vi "HEWH Get SUf Index.vi"(7 "Water Heater Type":T6, 8 "error in (no error)":errorcluster, 11 "UEF Calculated Values":T1={"Calculated Values"={"Draw Cluster - Actual (Gal)"=[], "Mass of water All (lbm)"=[], "Density of hot water All (lbm/gal)"=[], "CpHW (BTU/(lbm °F))"=[], "rho 2 (lb/gal)"=0.0, "rho standby (lb/gal)"=0.0, "rho 24 (lb/gal)"=0.0, "Cp1 (BTU/(lb*F))"=0.0, "Cp2 (BTU/(lb*F))"=0.0, "Cp standby (BTU/(lb*F))"=0.0, "Cp 24 (BTU/(lb*F))"=0.0, "nu_r"=0.0, "Qstby (BTU)"=0.0, "Qhr (BTU/hr)"=0.0, "UA (BTU/(hr*F))"=0.0, "Q (BTU)"=0.0, "Qd (BTU)"=0.0, "Qda (BTU)"=0.0, "QHW67 (BTU)"=0.0, "UEF"=0.0, "Tdel1-Mean Outlet 1st Cluster(°F)"=0.0, "Tin1 - Mean Inlet 1st Cluster (°F)"=0.0, "Cp theoretical (BTU/(lbm °F))"=0.0, "M cluster mass removed (lb)"=0.0, "V1- Vol (Gal)"=0.0, "Test Data -Start to End (Full Index)"=[], "rho_nu (lb/gal)"=0.0, "Density of cold water All (lbm/gal)"=[], "CpUEF (BTU/(lb*F))"=0.0, "QHW (BTU)"=0.0, "QHWD (BTU)"=0.0, "Qdm (BTU)"=0.0, "FHD-After 1 Hour (String)"=[], "Vn"=0.0, "T*avg_del(n)"=0.0, "Max Location"=0, "T*min(n-1)"=0.0, "T*avg_del(n-1)"=0.0, "Temp Greater than T*min(n-1)"=FALSE, "Adjustment Factor"=0.0, "Draw Bonus Volume (gal)"=0.0, "Flow Type - End Condition"=enum."ForcedDrawAfterHour"}, "Sampled Data"={"Cold Water Draw Amounts-(Gal)"=[14.98, 1.97, 9.0, 8.97, 4.98, 0.98, 0.96, 0.96, 0.96, 1.96, 1.99, 6.98], "T del_all - Outlet Temps (°F)"=[121.5, 121.3, 124.5, 120.0, 121.2, 120.1, 119.0, 120.3, 116.6, 118.8, 118.3, 118.3], "T in_all - Inlet Temps (°F)"=[58.5, 58.2, 58.4, 58.6, 58.6, 58.1, 58.1, 58.3, 56.3, 58.5, 58.5, 58.5], "Qsu0 (BTU)"=9772.3, "Qsuf (BTU)"=9773.0, "Tau stby_1 (hr)"=6.7, "T suf(°F)"=107.7, "T su0(°F)"=109.3, "T tstby(°F)"=108.5, "T astby(°F)"=68.2, "T 24(°F)"=117.9, "Qr (BTU)"=7628.5, "T0 (°F)"=121.1, "Tmax1 (°F)"=122.4, "Qe (BTU)"=29606.3, "Qf (BTU)"=0.0, "Tastby2 (°F)"=68.3, "RTD Out Full Data\nSet (Each Draw)"=[], "RTD IN Full Data\nSet (Each Draw)"=[], "Tau stby2 (hr)"=23.406, "Hot Water Draw Amounts-(Gal)"=[], "Cold Flow Rate (GPM)"=[], "Hot Flow Rate (GPM)"=[], "Softw Elapsed Time\n Full Data Set (Each Draw)"=[], "Cold Gal Total Full\nData Set (Each Draw)"=[], "Total Hot Draw Amount (Gal) "=0.0, "Total Cold Draw Amount (Gal)"=0.0, "Qe (Wh)"=0.0, "Hot Gal Total Full\nData Set (Each Draw)"=[]}, "Static Data"={"T-Wh Setpoint (°F)"=125.0, "T-Inlet Setpoint (°F)"=58.0, "T-Ambinet Nominal (°F)"=67.5, "V - Volume of Wh (True)"=46.0}, "Data Indexes"={"Test Start-Full Index (Found)"=0, "Header Length"=0, "Draw Index (Found)"=[], "Nr"=0, "Start Watt Hours"=0.0, "Tsu0 Index (Found)"=0, "Tsf Index (Found)"=0, "Start Energy (BTU-Gas)"=0.0, "Draws in Cluster"=0, "T0 Index-Full Index (Found)"=0, "Non-Draw Index (Found)"=[], "Tmax1 Index (Found)"=0, "Test End-Full Index (Found)"=0, "Heating Index (Found)"=[], "Heating Timestamp"=[], "Non-Draw Timestamp"=[], "Draw Index Timestamp"=[], "Tmax1 Timestamp"=0.0, "Tsu0 Timestamp"=0.0, "Tsf Timestamp"=0.0, "T0 Timestamp"=0.0, "Test End Timestamp"=0.0, "Test Start Timestamp"=0.0, "15 sec after Draw Timestamp"=[], "15 sec after Draw Index"=[], "Tmax1 Occurred During a Draw"=FALSE, "FHD Total Time (Sec)"=0.0, "Draw Pattern"=enum."Very Small Usage", "Standby Valid"=FALSE}, "Raw Data"={"Elapsed Time Index (DBL)"=0, "Software Elapsed Time Index (DBL)"=0, "TC Tree Avg Index (DBL)"=0, "Watt Hours -Wh Index (DBL)"=0, "Energy BTU Index (DBL)"=0, "Totalized Flow Index (DBL)"=0, "Flow Rate Index (DBL)"=0, "Program Status Index (Str)"=0, "RTDin Index (DBL)"=0, "RTDout Index (DBL)"=0, "RTDamb Index (DBL)"=0, "Test Data-Start to End DBL"=[], "Data Type"=enum."GEA Inlet Side Meter", "Heat Source Index (DBL)"=0, "Hot Water Rate GPM (DBL)"=0, "Hot Water Total - GAL (DBL)"=0, "FHD-After 1 hour"=[], "Humidity -% RH (DBL)"=0, "Voltage - V (DBL)"=0, "Draw Count (DBL)"=0, "Elapsed Time Index (Str)"=0, "Software Elapsed Time Index (Str)"=0, "Frequency-Hz (Str)"=0, "RTDin Index (Str)"=0, "RTDout Index (Str)"=0, "RTDamb Index (Str)"=0, "UE (Str)"=0, "LE (Str)"=0, "Compressor (Str)"=0, "Flow Rate Index (Str)"=0, "Hot Water Total - GAL (Str)"=0}, "Tolerance Check (T)=Pass"={"Flow Rate"=FALSE, "Totalized Flow"=FALSE, "Ambient Temp (Full Range)"=FALSE, "Ambient Humidity (Full Range)"=FALSE, "Inlet Temp"=FALSE, "Outlet Temp"=FALSE, "Valid Test"=FALSE, "Individual Totalized Flow"=FALSE, "Data Sheet Check"="", "Inlet Temperature"=[], "Tinlet Max"=[], "Tinlet Min"=[], "Flow Rate Max (Tol)"=[], "Flow Rate Min (Tol)"=[], "Amb Temp Max"=0.0, "Amb Temp Min"=0.0, "Toutlet Max - Draw 1"=0.0, "Humidity Upper Tolerance (%)"=0.0, "Total Volume Tolerance (Gal)"=0.0, "Humidity Lower Tolerance (%)"=0.0, "Flow Rate Max\nPer Draw"=[], "Flow Rate Min\nPer Draw"=[], "Ambient Humidity (Runtime)"=FALSE, "Humidity Avg (Runtime)"=0.0, "Ambient Temp (On-Time AVG)"=FALSE, "Ambient Temp (Off-Time AVG)"=FALSE, "Amb Temp OFF Avg"=0.0, "Amb Temp ON Avg"=0.0, "Voltage (Heating)"=FALSE, "Voltage (Min)"=0.0, "Voltage (Max)"=0.0, "Toutlet Max"=[], "Toutlet Min"=[]}, "Test Information"={"TR Number"="", "Lab ID"="", "Notes/Config"="", "Model Number"="", "Serial Number"="", "Lab Technician"="", "Engineer"="", "Type of Fuel"="", "Samp Received Date"="", "Samp Test Date"="", "Report Date"="", "Rate Input (kW or BTU/hr)"="", "Measured Input (kW or BTU/hr)"="", "Filename"="", "Calibration Information"=[], "Calculator Version"="", "Minimum UEF Per CFR"=0.0, "UEF Report Information"=[], "FHR Report Information"=[], "FHR Front Panel Display"=[], "UEF Front Panel Display"=[], "Draw Outlet Temp Viewer"=[]}} {"Data Indexes"."15 sec after Draw Index" format="%#.2f"; "Data Indexes"."15 sec after Draw Timestamp" format="%#.2f"; "Data Indexes"."Test Start Timestamp" format="%.2f"; "Data Indexes"."Test End Timestamp" format="%.2f"; "Data Indexes"."T0 Timestamp" format="%.2f"; "Data Indexes"."Tsf Timestamp" format="%.2f"; "Data Indexes"."Tsu0 Timestamp" format="%.2f"; "Data Indexes"."Tmax1 Timestamp" format="%.2f"; "Data Indexes"."Draw Index Timestamp" format="%#.2f"; "Data Indexes"."Non-Draw Timestamp" format="%#.2f"; "Data Indexes"."Heating Timestamp" format="%#.2f"; "Data Indexes"."Start Energy (BTU-Gas)" format="%.6f"; "Data Indexes"."Start Watt Hours" format="%.6f"; "Static Data"."V - Volume of Wh (True)" format="%.5f"; "Static Data"."T-Ambinet Nominal (°F)" format="%.5f"; "Static Data"."T-Inlet Setpoint (°F)" format="%.5f"; "Static Data"."T-Wh Setpoint (°F)" format="%.5f"; "Sampled Data"."Qe (Wh)" format="%.5f"; "Sampled Data"."Tau stby2 (hr)" format="%.5f"; "Sampled Data"."Tastby2 (°F)" format="%.5f"; "Sampled Data"."Qf (BTU)" format="%.5f"; "Sampled Data"."Qe (BTU)" format="%.5f"; "Sampled Data"."Tmax1 (°F)" format="%.5f"; "Sampled Data"."T0 (°F)" format="%.5f"; "Sampled Data"."Qr (BTU)" format="%.5f"; "Sampled Data"."T 24(°F)" format="%.5f"; "Sampled Data"."T astby(°F)" format="%.5f"; "Sampled Data"."T tstby(°F)" format="%.5f"; "Sampled Data"."T su0(°F)" format="%.5f"; "Sampled Data"."T suf(°F)" format="%.5f"; "Sampled Data"."Tau stby_1 (hr)" format="%.5f"; "Sampled Data"."Qsuf (BTU)" format="%.5f"; "Sampled Data"."Qsu0 (BTU)" format="%.5f"; "Calculated Values"."Draw Bonus Volume (gal)" format="%.6f"; "Calculated Values"."Adjustment Factor" format="%.6f"; "Calculated Values"."T*avg_del(n-1)" format="%.6f"; "Calculated Values"."T*min(n-1)" format="%.6f"; "Calculated Values"."T*avg_del(n)" format="%.6f"; "Calculated Values"."Vn" format="%.6f"; "Calculated Values"."Qdm (BTU)" format="%.6f"; "Calculated Values"."QHWD (BTU)" format="%.6f"; "Calculated Values"."QHW (BTU)" format="%.6f"; "Calculated Values"."UEF" format="%.6f"; "Calculated Values"."QHW67 (BTU)" format="%.6f"; "Calculated Values"."Qda (BTU)" format="%.6f"; "Calculated Values"."Qd (BTU)" format="%.6f"; "Calculated Values"."Q (BTU)" format="%.6f"; "Calculated Values"."UA (BTU/(hr*F))" format="%.6f"; "Calculated Values"."Qhr (BTU/hr)" format="%.6f"; "Calculated Values"."Qstby (BTU)" format="%.6f"; "Calculated Values"."nu_r" format="%.6f"; "Calculated Values"."CpUEF (BTU/(lb*F))" format="%.6f"; "Calculated Values"."rho_nu (lb/gal)" format="%.6f"; "Calculated Values"."V1- Vol (Gal)" format="%.6f"; "Calculated Values"."M cluster mass removed (lb)" format="%.6f"; "Calculated Values"."Cp theoretical (BTU/(lbm °F))" format="%.6f"; "Calculated Values"."Tin1 - Mean Inlet 1st Cluster (°F)" format="%.6f"; "Calculated Values"."Tdel1-Mean Outlet 1st Cluster(°F)" format="%.6f"; "Calculated Values"."Cp 24 (BTU/(lb*F))" format="%.6f"; "Calculated Values"."Cp standby (BTU/(lb*F))" format="%.6f"; "Calculated Values"."Cp2 (BTU/(lb*F))" format="%.6f"; "Calculated Values"."Cp1 (BTU/(lb*F))" format="%.6f"; "Calculated Values"."rho 24 (lb/gal)" format="%.6f"; "Calculated Values"."rho standby (lb/gal)" format="%.6f"; "Calculated Values"."rho 2 (lb/gal)" format="%.6f"; "Calculated Values"."Density of cold water All (lbm/gal)" format="%#.3g"; "Calculated Values"."CpHW (BTU/(lbm °F))" format="%#.3g"; "Calculated Values"."Density of hot water All (lbm/gal)" format="%#.3g"; "Calculated Values"."Mass of water All (lbm)" format="%#.3f"}) -> (0 "error out":errorcluster, 3 "UEF Calculated Values Output":T1={"Calculated Values"={"Draw Cluster - Actual (Gal)"=[], "Mass of water All (lbm)"=[], "Density of hot water All (lbm/gal)"=[], "CpHW (BTU/(lbm °F))"=[], "rho 2 (lb/gal)"=0.0, "rho standby (lb/gal)"=0.0, "rho 24 (lb/gal)"=0.0, "Cp1 (BTU/(lb*F))"=0.0, "Cp2 (BTU/(lb*F))"=0.0, "Cp standby (BTU/(lb*F))"=0.0, "Cp 24 (BTU/(lb*F))"=0.0, "nu_r"=0.0, "Qstby (BTU)"=0.0, "Qhr (BTU/hr)"=0.0, "UA (BTU/(hr*F))"=0.0, "Q (BTU)"=0.0, "Qd (BTU)"=0.0, "Qda (BTU)"=0.0, "QHW67 (BTU)"=0.0, "UEF"=0.0, "Tdel1-Mean Outlet 1st Cluster(°F)"=0.0, "Tin1 - Mean Inlet 1st Cluster (°F)"=0.0, "Cp theoretical (BTU/(lbm °F))"=0.0, "M cluster mass removed (lb)"=0.0, "V1- Vol (Gal)"=0.0, "Test Data -Start to End (Full Index)"=[], "rho_nu (lb/gal)"=0.0, "Density of cold water All (lbm/gal)"=[], "CpUEF (BTU/(lb*F))"=0.0, "QHW (BTU)"=0.0, "QHWD (BTU)"=0.0, "Qdm (BTU)"=0.0, "FHD-After 1 Hour (String)"=[], "Vn"=0.0, "T*avg_del(n)"=0.0, "Max Location"=0, "T*min(n-1)"=0.0, "T*avg_del(n-1)"=0.0, "Temp Greater than T*min(n-1)"=FALSE, "Adjustment Factor"=0.0, "Draw Bonus Volume (gal)"=0.0, "Flow Type - End Condition"=enum."ForcedDrawAfterHour"}, "Sampled Data"={"Cold Water Draw Amounts-(Gal)"=[14.98, 1.97, 9.0, 8.97, 4.98, 0.98, 0.96, 0.96, 0.96, 1.96, 1.99, 6.98], "T del_all - Outlet Temps (°F)"=[121.5, 121.3, 124.5, 120.0, 121.2, 120.1, 119.0, 120.3, 116.6, 118.8, 118.3, 118.3], "T in_all - Inlet Temps (°F)"=[58.5, 58.2, 58.4, 58.6, 58.6, 58.1, 58.1, 58.3, 56.3, 58.5, 58.5, 58.5], "Qsu0 (BTU)"=9772.3, "Qsuf (BTU)"=9773.0, "Tau stby_1 (hr)"=6.7, "T suf(°F)"=107.7, "T su0(°F)"=109.3, "T tstby(°F)"=108.5, "T astby(°F)"=68.2, "T 24(°F)"=117.9, "Qr (BTU)"=7628.5, "T0 (°F)"=121.1, "Tmax1 (°F)"=122.4, "Qe (BTU)"=29606.3, "Qf (BTU)"=0.0, "Tastby2 (°F)"=68.3, "RTD Out Full Data\nSet (Each Draw)"=[], "RTD IN Full Data\nSet (Each Draw)"=[], "Tau stby2 (hr)"=23.406, "Hot Water Draw Amounts-(Gal)"=[], "Cold Flow Rate (GPM)"=[], "Hot Flow Rate (GPM)"=[], "Softw Elapsed Time\n Full Data Set (Each Draw)"=[], "Cold Gal Total Full\nData Set (Each Draw)"=[], "Total Hot Draw Amount (Gal) "=0.0, "Total Cold Draw Amount (Gal)"=0.0, "Qe (Wh)"=0.0, "Hot Gal Total Full\nData Set (Each Draw)"=[]}, "Static Data"={"T-Wh Setpoint (°F)"=125.0, "T-Inlet Setpoint (°F)"=58.0, "T-Ambinet Nominal (°F)"=67.5, "V - Volume of Wh (True)"=46.0}, "Data Indexes"={"Test Start-Full Index (Found)"=0, "Header Length"=0, "Draw Index (Found)"=[], "Nr"=0, "Start Watt Hours"=0.0, "Tsu0 Index (Found)"=0, "Tsf Index (Found)"=0, "Start Energy (BTU-Gas)"=0.0, "Draws in Cluster"=0, "T0 Index-Full Index (Found)"=0, "Non-Draw Index (Found)"=[], "Tmax1 Index (Found)"=0, "Test End-Full Index (Found)"=0, "Heating Index (Found)"=[], "Heating Timestamp"=[], "Non-Draw Timestamp"=[], "Draw Index Timestamp"=[], "Tmax1 Timestamp"=0.0, "Tsu0 Timestamp"=0.0, "Tsf Timestamp"=0.0, "T0 Timestamp"=0.0, "Test End Timestamp"=0.0, "Test Start Timestamp"=0.0, "15 sec after Draw Timestamp"=[], "15 sec after Draw Index"=[], "Tmax1 Occurred During a Draw"=FALSE, "FHD Total Time (Sec)"=0.0, "Draw Pattern"=enum."Very Small Usage", "Standby Valid"=FALSE}, "Raw Data"={"Elapsed Time Index (DBL)"=0, "Software Elapsed Time Index (DBL)"=0, "TC Tree Avg Index (DBL)"=0, "Watt Hours -Wh Index (DBL)"=0, "Energy BTU Index (DBL)"=0, "Totalized Flow Index (DBL)"=0, "Flow Rate Index (DBL)"=0, "Program Status Index (Str)"=0, "RTDin Index (DBL)"=0, "RTDout Index (DBL)"=0, "RTDamb Index (DBL)"=0, "Test Data-Start to End DBL"=[], "Data Type"=enum."GEA Inlet Side Meter", "Heat Source Index (DBL)"=0, "Hot Water Rate GPM (DBL)"=0, "Hot Water Total - GAL (DBL)"=0, "FHD-After 1 hour"=[], "Humidity -% RH (DBL)"=0, "Voltage - V (DBL)"=0, "Draw Count (DBL)"=0, "Elapsed Time Index (Str)"=0, "Software Elapsed Time Index (Str)"=0, "Frequency-Hz (Str)"=0, "RTDin Index (Str)"=0, "RTDout Index (Str)"=0, "RTDamb Index (Str)"=0, "UE (Str)"=0, "LE (Str)"=0, "Compressor (Str)"=0, "Flow Rate Index (Str)"=0, "Hot Water Total - GAL (Str)"=0}, "Tolerance Check (T)=Pass"={"Flow Rate"=FALSE, "Totalized Flow"=FALSE, "Ambient Temp (Full Range)"=FALSE, "Ambient Humidity (Full Range)"=FALSE, "Inlet Temp"=FALSE, "Outlet Temp"=FALSE, "Valid Test"=FALSE, "Individual Totalized Flow"=FALSE, "Data Sheet Check"="", "Inlet Temperature"=[], "Tinlet Max"=[], "Tinlet Min"=[], "Flow Rate Max (Tol)"=[], "Flow Rate Min (Tol)"=[], "Amb Temp Max"=0.0, "Amb Temp Min"=0.0, "Toutlet Max - Draw 1"=0.0, "Humidity Upper Tolerance (%)"=0.0, "Total Volume Tolerance (Gal)"=0.0, "Humidity Lower Tolerance (%)"=0.0, "Flow Rate Max\nPer Draw"=[], "Flow Rate Min\nPer Draw"=[], "Ambient Humidity (Runtime)"=FALSE, "Humidity Avg (Runtime)"=0.0, "Ambient Temp (On-Time AVG)"=FALSE, "Ambient Temp (Off-Time AVG)"=FALSE, "Amb Temp OFF Avg"=0.0, "Amb Temp ON Avg"=0.0, "Voltage (Heating)"=FALSE, "Voltage (Min)"=0.0, "Voltage (Max)"=0.0, "Toutlet Max"=[], "Toutlet Min"=[]}, "Test Information"={"TR Number"="", "Lab ID"="", "Notes/Config"="", "Model Number"="", "Serial Number"="", "Lab Technician"="", "Engineer"="", "Type of Fuel"="", "Samp Received Date"="", "Samp Test Date"="", "Report Date"="", "Rate Input (kW or BTU/hr)"="", "Measured Input (kW or BTU/hr)"="", "Filename"="", "Calibration Information"=[], "Calculator Version"="", "Minimum UEF Per CFR"=0.0, "UEF Report Information"=[], "FHR Report Information"=[], "FHR Front Panel Display"=[], "UEF Front Panel Display"=[], "Draw Outlet Temp Viewer"=[]}} {"Data Indexes"."15 sec after Draw Index" format="%#.2f"; "Data Indexes"."15 sec after Draw Timestamp" format="%#.2f"; "Data Indexes"."Test Start Timestamp" format="%.2f"; "Data Indexes"."Test End Timestamp" format="%.2f"; "Data Indexes"."T0 Timestamp" format="%.2f"; "Data Indexes"."Tsf Timestamp" format="%.2f"; "Data Indexes"."Tsu0 Timestamp" format="%.2f"; "Data Indexes"."Tmax1 Timestamp" format="%.2f"; "Data Indexes"."Draw Index Timestamp" format="%#.2f"; "Data Indexes"."Non-Draw Timestamp" format="%#.2f"; "Data Indexes"."Heating Timestamp" format="%#.2f"; "Data Indexes"."Start Energy (BTU-Gas)" format="%.6f"; "Data Indexes"."Start Watt Hours" format="%.6f"; "Static Data"."V - Volume of Wh (True)" format="%.5f"; "Static Data"."T-Ambinet Nominal (°F)" format="%.5f"; "Static Data"."T-Inlet Setpoint (°F)" format="%.5f"; "Static Data"."T-Wh Setpoint (°F)" format="%.5f"; "Sampled Data"."Qe (Wh)" format="%.5f"; "Sampled Data"."Tau stby2 (hr)" format="%.5f"; "Sampled Data"."Tastby2 (°F)" format="%.5f"; "Sampled Data"."Qf (BTU)" format="%.5f"; "Sampled Data"."Qe (BTU)" format="%.5f"; "Sampled Data"."Tmax1 (°F)" format="%.5f"; "Sampled Data"."T0 (°F)" format="%.5f"; "Sampled Data"."Qr (BTU)" format="%.5f"; "Sampled Data"."T 24(°F)" format="%.5f"; "Sampled Data"."T astby(°F)" format="%.5f"; "Sampled Data"."T tstby(°F)" format="%.5f"; "Sampled Data"."T su0(°F)" format="%.5f"; "Sampled Data"."T suf(°F)" format="%.5f"; "Sampled Data"."Tau stby_1 (hr)" format="%.5f"; "Sampled Data"."Qsuf (BTU)" format="%.5f"; "Sampled Data"."Qsu0 (BTU)" format="%.5f"; "Calculated Values"."Draw Bonus Volume (gal)" format="%.6f"; "Calculated Values"."Adjustment Factor" format="%.6f"; "Calculated Values"."T*avg_del(n-1)" format="%.6f"; "Calculated Values"."T*min(n-1)" format="%.6f"; "Calculated Values"."T*avg_del(n)" format="%.6f"; "Calculated Values"."Vn" format="%.6f"; "Calculated Values"."Qdm (BTU)" format="%.6f"; "Calculated Values"."QHWD (BTU)" format="%.6f"; "Calculated Values"."QHW (BTU)" format="%.6f"; "Calculated Values"."UEF" format="%.6f"; "Calculated Values"."QHW67 (BTU)" format="%.6f"; "Calculated Values"."Qda (BTU)" format="%.6f"; "Calculated Values"."Qd (BTU)" format="%.6f"; "Calculated Values"."Q (BTU)" format="%.6f"; "Calculated Values"."UA (BTU/(hr*F))" format="%.6f"; "Calculated Values"."Qhr (BTU/hr)" format="%.6f"; "Calculated Values"."Qstby (BTU)" format="%.6f"; "Calculated Values"."nu_r" format="%.6f"; "Calculated Values"."CpUEF (BTU/(lb*F))" format="%.6f"; "Calculated Values"."rho_nu (lb/gal)" format="%.6f"; "Calculated Values"."V1- Vol (Gal)" format="%.6f"; "Calculated Values"."M cluster mass removed (lb)" format="%.6f"; "Calculated Values"."Cp theoretical (BTU/(lbm °F))" format="%.6f"; "Calculated Values"."Tin1 - Mean Inlet 1st Cluster (°F)" format="%.6f"; "Calculated Values"."Tdel1-Mean Outlet 1st Cluster(°F)" format="%.6f"; "Calculated Values"."Cp 24 (BTU/(lb*F))" format="%.6f"; "Calculated Values"."Cp standby (BTU/(lb*F))" format="%.6f"; "Calculated Values"."Cp2 (BTU/(lb*F))" format="%.6f"; "Calculated Values"."Cp1 (BTU/(lb*F))" format="%.6f"; "Calculated Values"."rho 24 (lb/gal)" format="%.6f"; "Calculated Values"."rho standby (lb/gal)" format="%.6f"; "Calculated Values"."rho 2 (lb/gal)" format="%.6f"; "Calculated Values"."Density of cold water All (lbm/gal)" format="%#.3g"; "Calculated Values"."CpHW (BTU/(lbm °F))" format="%#.3g"; "Calculated Values"."Density of hot water All (lbm/gal)" format="%#.3g"; "Calculated Values"."Mass of water All (lbm)" format="%#.3f"})   [LabVIEW 2023]
uses:
  Type Definitions/UEF Constants.ctl
  Type Definitions/HEWH Draw Stats.ctl
  Type Definitions/HEWH FHR Draw Type.ctl
  Type Definitions/FHR Bins.ctl
  Type Definitions/HEWH Meter Type.ctl
  Type Definitions/HEWH Water Heater Type.ctl
panel:
  # "FHR"
  # "FHR"
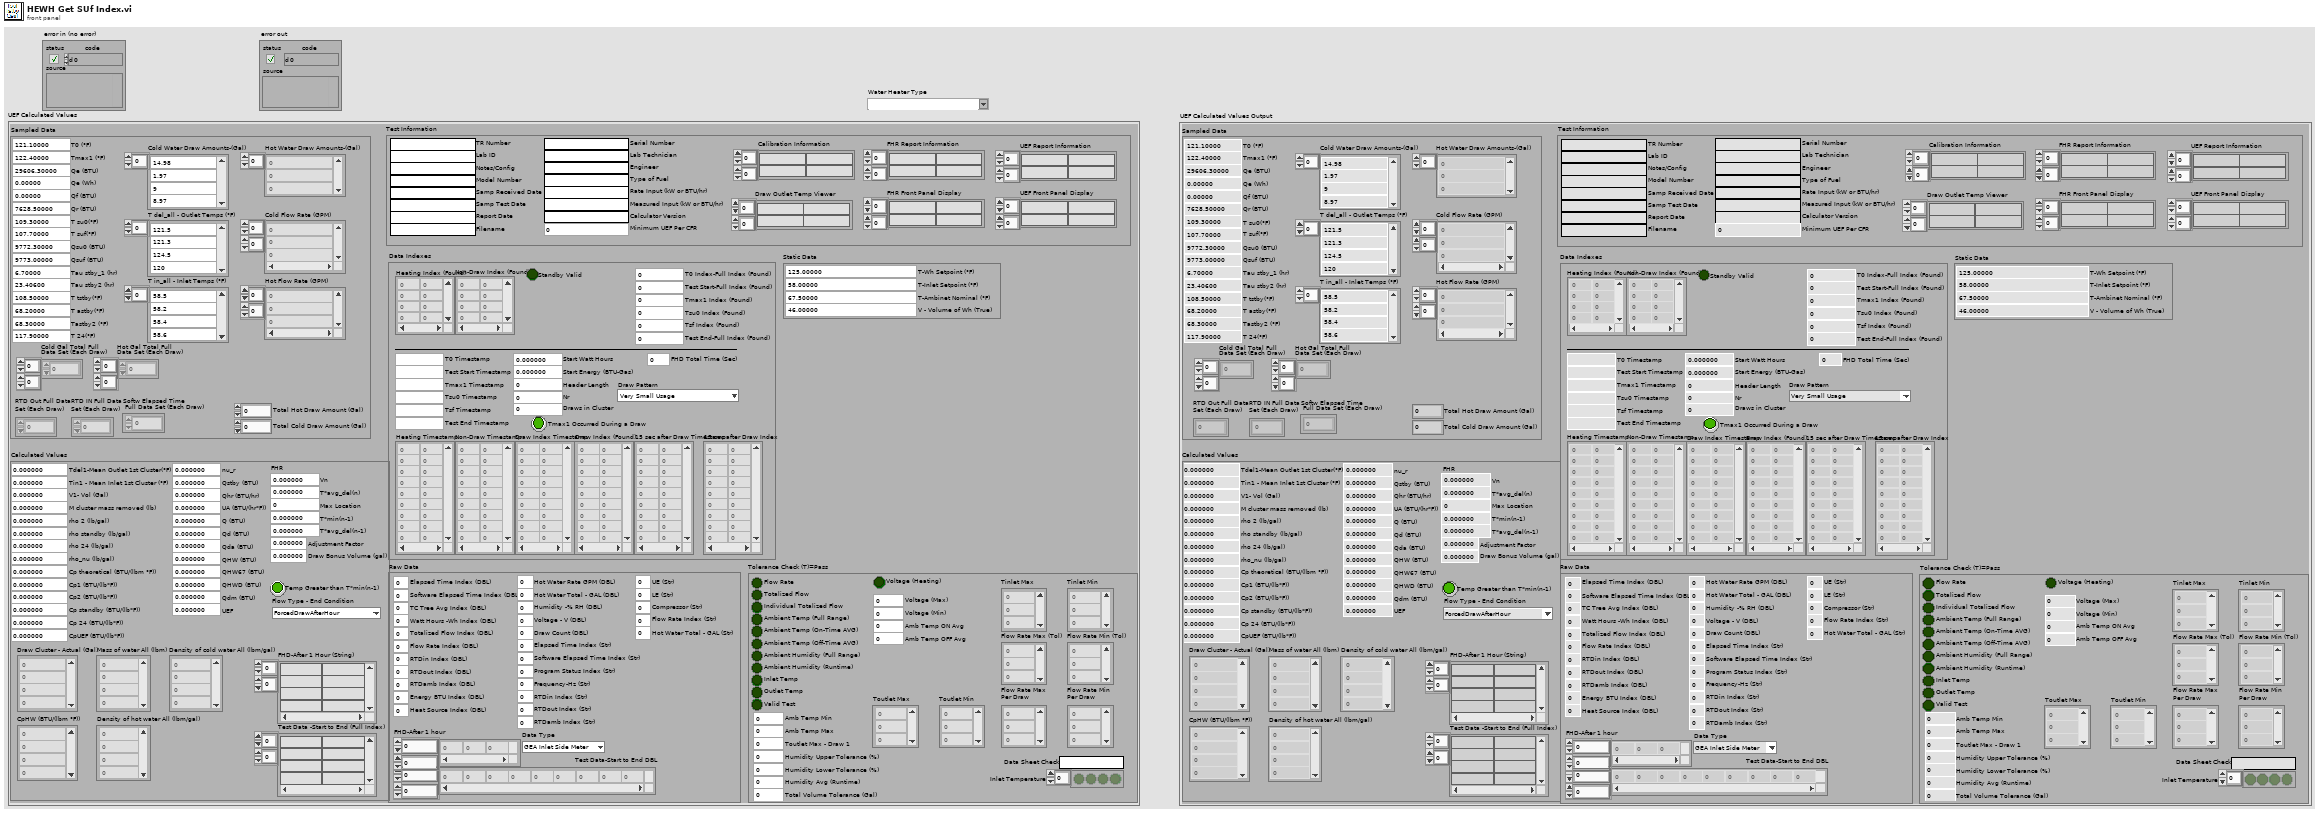
[diagram p1: front panel]
types:
  T1 = typedef "UEF Constants.ctl" = cluster{"Calculated Values":T2, "Sampled Data":cluster{"Cold Water Draw Amounts-(Gal)":dbl[], "T del_all - Outlet Temps (°F)":dbl[], "T in_all - Inlet Temps (°F)":dbl[], "Qsu0 (BTU)":dbl, "Qsuf (BTU)":dbl, "Tau stby_1 (hr)":dbl, "T suf(°F)":dbl, "T su0(°F)":dbl, "T tstby(°F)":dbl, "T astby(°F)":dbl, "T 24(°F)":dbl, "Qr (BTU)":dbl, "T0 (°F)":dbl, "Tmax1 (°F)":dbl, "Qe (BTU)":dbl, "Qf (BTU)":dbl, "Tastby2 (°F)":dbl, "RTD Out Full Data\nSet (Each Draw)":dbl[][], "RTD IN Full Data\nSet (Each Draw)":dbl[][], "Tau stby2 (hr)":dbl, "Hot Water Draw Amounts-(Gal)":dbl[], "Cold Flow Rate (GPM)":dbl[][], "Hot Flow Rate (GPM)":dbl[][], "Softw Elapsed Time\n Full Data Set (Each Draw)":dbl[][], "Cold Gal Total Full\nData Set (Each Draw)":dbl[][], "Total Hot Draw Amount (Gal) ":dbl, "Total Cold Draw Amount (Gal)":dbl, "Qe (Wh)":dbl, "Hot Gal Total Full\nData Set (Each Draw)":dbl[][]}, "Static Data":cluster{"T-Wh Setpoint (°F)":dbl, "T-Inlet Setpoint (°F)":dbl, "T-Ambinet Nominal (°F)":dbl, "V - Volume of Wh (True)":dbl}, "Data Indexes":cluster{"Test Start-Full Index (Found)":i32, "Header Length":i32, "Draw Index (Found)":i32[][], "Nr":i32, "Start Watt Hours":dbl, "Tsu0 Index (Found)":i32, "Tsf Index (Found)":i32, "Start Energy (BTU-Gas)":dbl, "Draws in Cluster":i32, "T0 Index-Full Index (Found)":i32, "Non-Draw Index (Found)":i32[][], "Tmax1 Index (Found)":i32, "Test End-Full Index (Found)":i32, "Heating Index (Found)":i32[][], "Heating Timestamp":dbl[][], "Non-Draw Timestamp":dbl[][], "Draw Index Timestamp":dbl[][], "Tmax1 Timestamp":dbl, "Tsu0 Timestamp":dbl, "Tsf Timestamp":dbl, "T0 Timestamp":dbl, "Test End Timestamp":dbl, "Test Start Timestamp":dbl, "15 sec after Draw Timestamp":dbl[][], "15 sec after Draw Index":dbl[][], "Tmax1 Occurred During a Draw":bool, "FHD Total Time (Sec)":dbl, "Draw Pattern":T4, "Standby Valid":bool}, "Raw Data":cluster{"Elapsed Time Index (DBL)":i32, "Software Elapsed Time Index (DBL)":i32, "TC Tree Avg Index (DBL)":i32, "Watt Hours -Wh Index (DBL)":i32, "Energy BTU Index (DBL)":i32, "Totalized Flow Index (DBL)":i32, "Flow Rate Index (DBL)":i32, "Program Status Index (Str)":i32, "RTDin Index (DBL)":i32, "RTDout Index (DBL)":i32, "RTDamb Index (DBL)":i32, "Test Data-Start to End DBL":dbl[][], "Data Type":T5, "Heat Source Index (DBL)":i32, "Hot Water Rate GPM (DBL)":i32, "Hot Water Total - GAL (DBL)":i32, "FHD-After 1 hour":dbl[][], "Humidity -% RH (DBL)":i32, "Voltage - V (DBL)":i32, "Draw Count (DBL)":i32, "Elapsed Time Index (Str)":i32, "Software Elapsed Time Index (Str)":i32, "Frequency-Hz (Str)":i32, "RTDin Index (Str)":i32, "RTDout Index (Str)":i32, "RTDamb Index (Str)":i32, "UE (Str)":i32, "LE (Str)":i32, "Compressor (Str)":i32, "Flow Rate Index (Str)":i32, "Hot Water Total - GAL (Str)":i32}, "Tolerance Check (T)=Pass":cluster{"Flow Rate":bool, "Totalized Flow":bool, "Ambient Temp (Full Range)":bool, "Ambient Humidity (Full Range)":bool, "Inlet Temp":bool, "Outlet Temp":bool, "Valid Test":bool, "Individual Totalized Flow":bool, "Data Sheet Check":string, "Inlet Temperature":bool[], "Tinlet Max":dbl[], "Tinlet Min":dbl[], "Flow Rate Max (Tol)":dbl[], "Flow Rate Min (Tol)":dbl[], "Amb Temp Max":dbl, "Amb Temp Min":dbl, "Toutlet Max - Draw 1":dbl, "Humidity Upper Tolerance (%)":dbl, "Total Volume Tolerance (Gal)":dbl, "Humidity Lower Tolerance (%)":dbl, "Flow Rate Max\nPer Draw":dbl[], "Flow Rate Min\nPer Draw":dbl[], "Ambient Humidity (Runtime)":bool, "Humidity Avg (Runtime)":dbl, "Ambient Temp (On-Time AVG)":bool, "Ambient Temp (Off-Time AVG)":bool, "Amb Temp OFF Avg":dbl, "Amb Temp ON Avg":dbl, "Voltage (Heating)":bool, "Voltage (Min)":dbl, "Voltage (Max)":dbl, "Toutlet Max":dbl[], "Toutlet Min":dbl[]}, "Test Information":cluster{"TR Number":string, "Lab ID":string, "Notes/Config":string, "Model Number":string, "Serial Number":string, "Lab Technician":string, "Engineer":string, "Type of Fuel":string, "Samp Received Date":string, "Samp Test Date":string, "Report Date":string, "Rate Input (kW or BTU/hr)":string, "Measured Input (kW or BTU/hr)":string, "Filename":string, "Calibration Information":string[][], "Calculator Version":string, "Minimum UEF Per CFR":dbl, "UEF Report Information":string[][], "FHR Report Information":string[][], "FHR Front Panel Display":string[][], "UEF Front Panel Display":string[][], "Draw Outlet Temp Viewer":string[][]}}
  T2 = typedef "HEWH Draw Stats.ctl" = cluster{"Draw Cluster - Actual (Gal)":dbl[], "Mass of water All (lbm)":dbl[], "Density of hot water All (lbm/gal)":dbl[], "CpHW (BTU/(lbm °F))":dbl[], "rho 2 (lb/gal)":dbl, "rho standby (lb/gal)":dbl, "rho 24 (lb/gal)":dbl, "Cp1 (BTU/(lb*F))":dbl, "Cp2 (BTU/(lb*F))":dbl, "Cp standby (BTU/(lb*F))":dbl, "Cp 24 (BTU/(lb*F))":dbl, "nu_r":dbl, "Qstby (BTU)":dbl, "Qhr (BTU/hr)":dbl, "UA (BTU/(hr*F))":dbl, "Q (BTU)":dbl, "Qd (BTU)":dbl, "Qda (BTU)":dbl, "QHW67 (BTU)":dbl, "UEF":dbl, "Tdel1-Mean Outlet 1st Cluster(°F)":dbl, "Tin1 - Mean Inlet 1st Cluster (°F)":dbl, "Cp theoretical (BTU/(lbm °F))":dbl, "M cluster mass removed (lb)":dbl, "V1- Vol (Gal)":dbl, "Test Data -Start to End (Full Index)":string[][], "rho_nu (lb/gal)":dbl, "Density of cold water All (lbm/gal)":dbl[], "CpUEF (BTU/(lb*F))":dbl, "QHW (BTU)":dbl, "QHWD (BTU)":dbl, "Qdm (BTU)":dbl, "FHD-After 1 Hour (String)":string[][], "Vn":dbl, "T*avg_del(n)":dbl, "Max Location":i32, "T*min(n-1)":dbl, "T*avg_del(n-1)":dbl, "Temp Greater than T*min(n-1)":bool, "Adjustment Factor":dbl, "Draw Bonus Volume (gal)":dbl, "Flow Type - End Condition":T3}
  T3 = typedef "HEWH FHR Draw Type.ctl" = enum16{"ForcedDrawAfterHour", "HeatingCutoffBeforeHour"}
  T4 = typedef "FHR Bins.ctl" = enum16{"Very Small Usage", "Low Usage", "Medium Usage", "High Usage", "Undefined"}
  T5 = typedef "HEWH Meter Type.ctl" = enum16{"GEA Inlet Side Meter", "GEA Outlet Side Meter", "CSA Inlet Side Meter"}
  T6 = typedef "HEWH Water Heater Type.ctl" = string
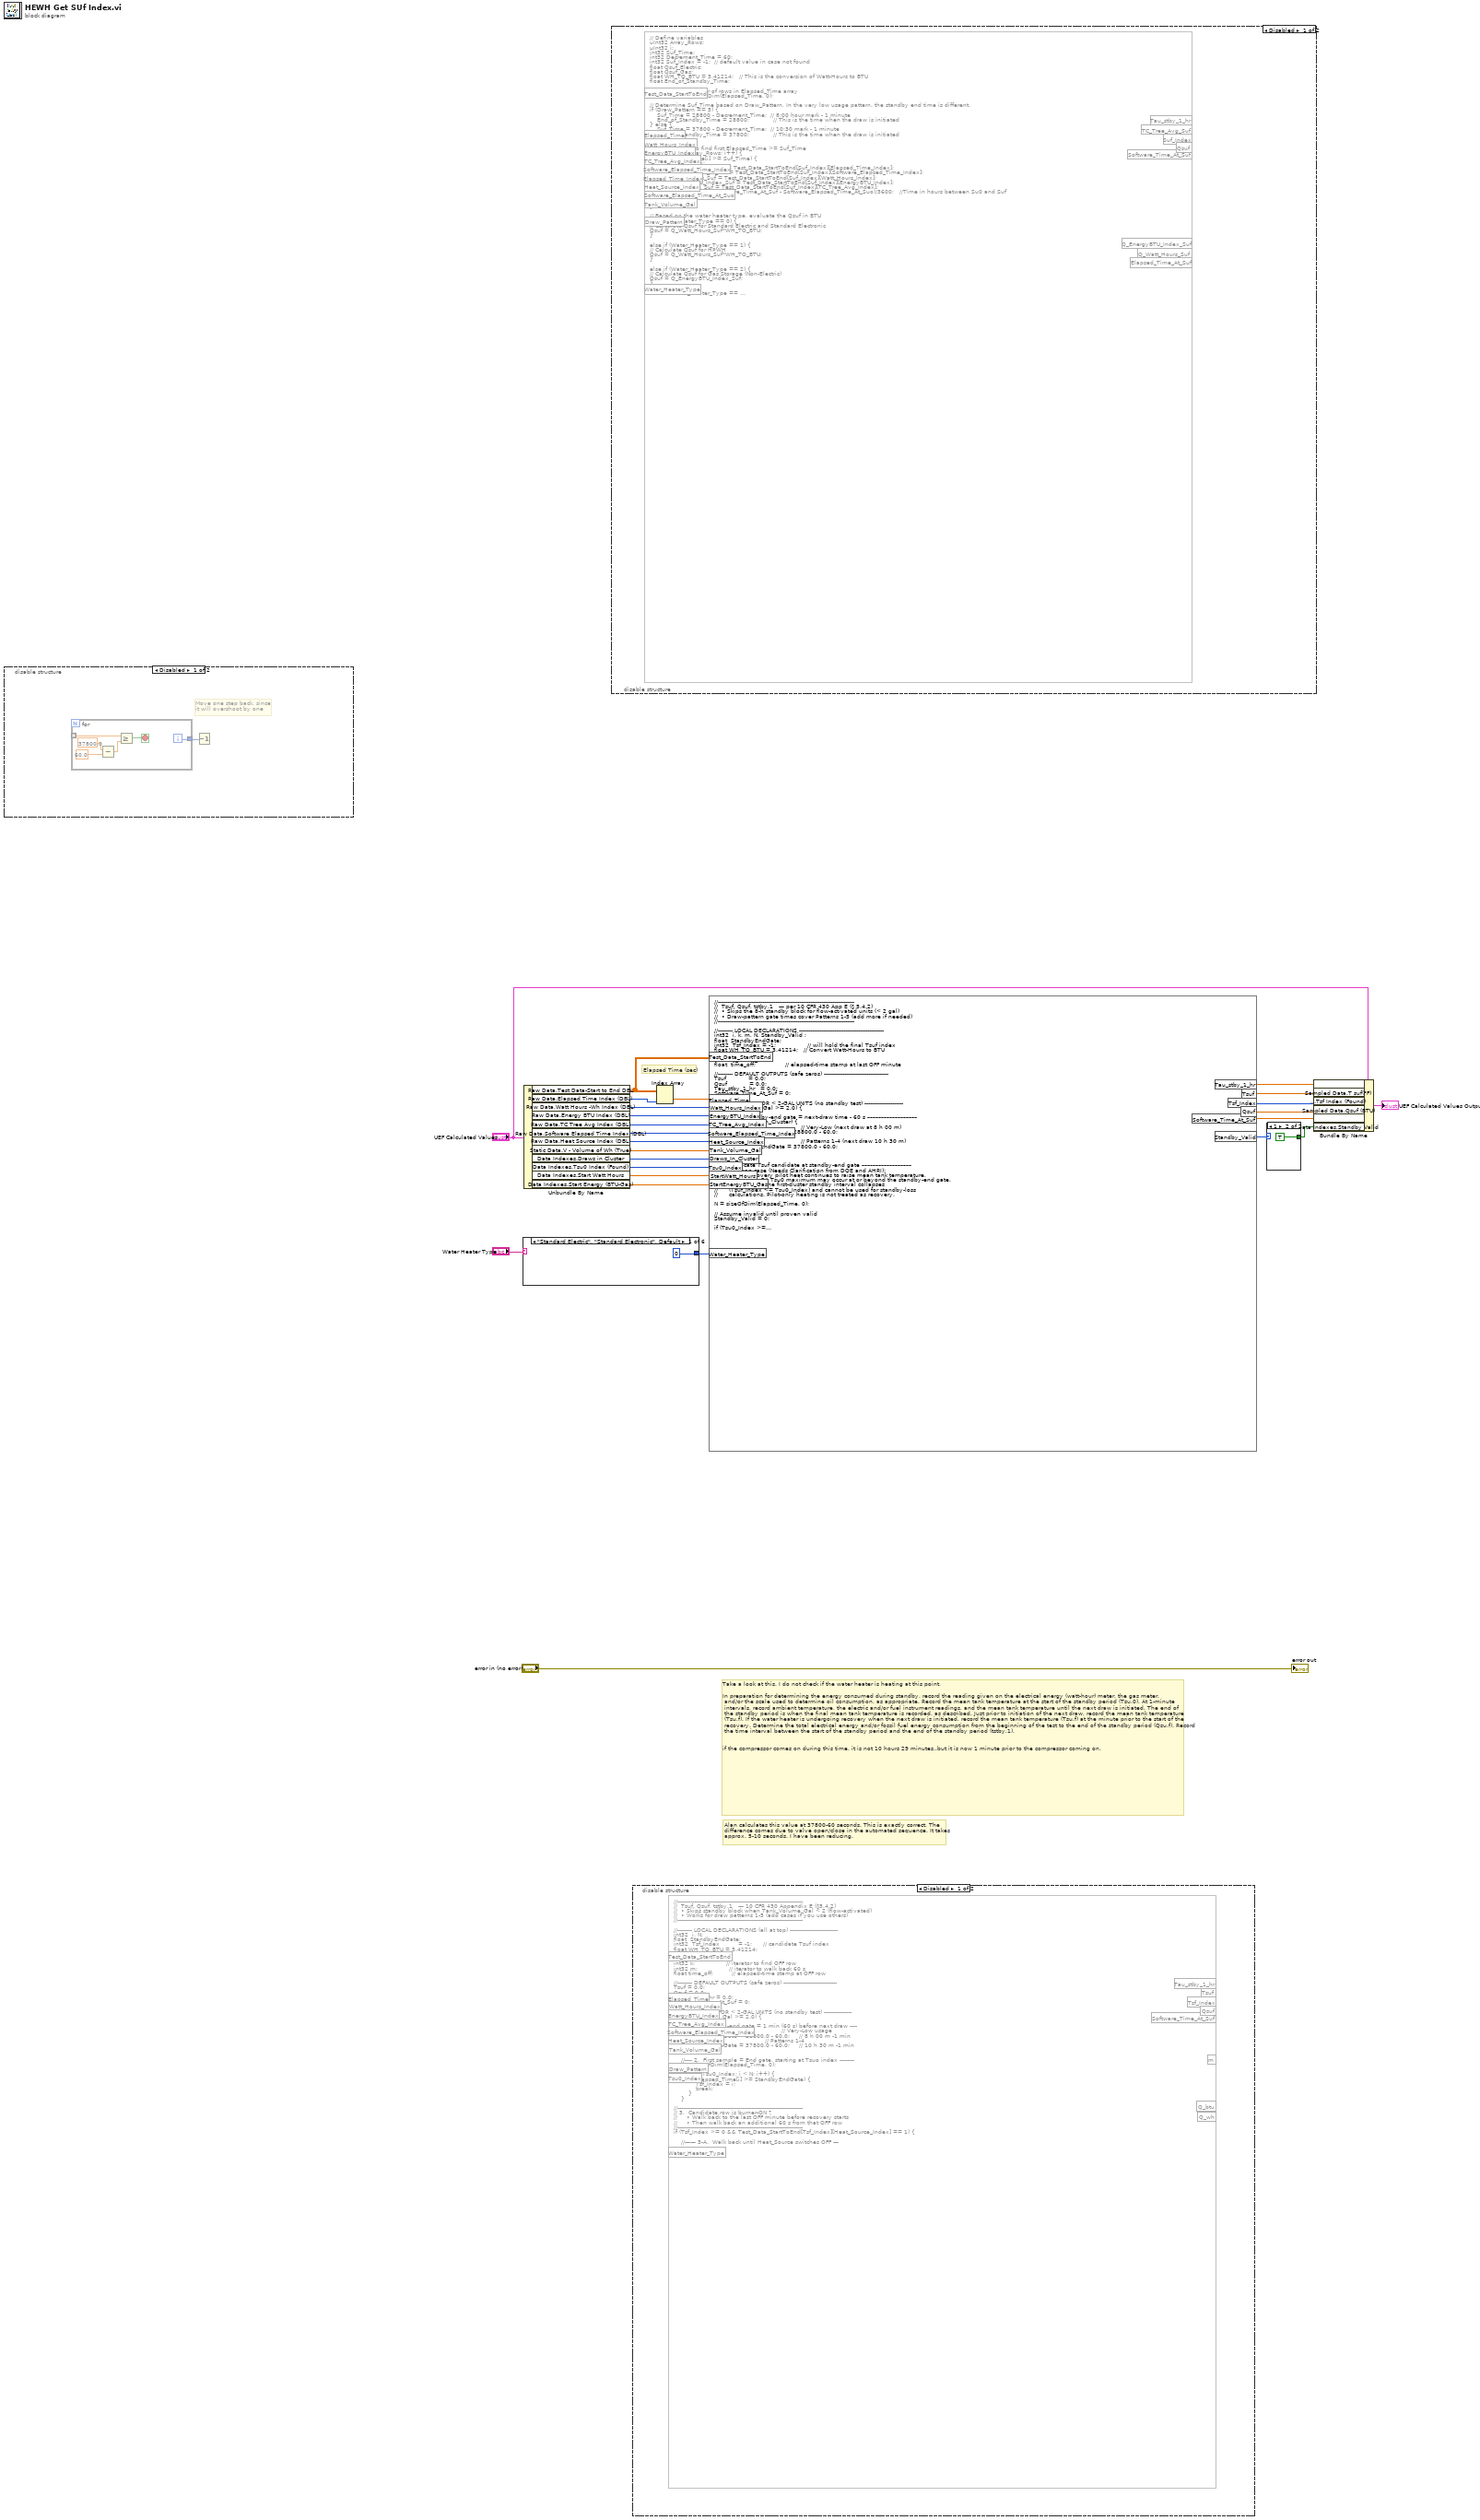
[diagram p0: block diagram]
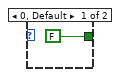
[diagram p2: hidden frame]
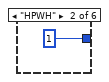
[diagram p5: hidden frame]
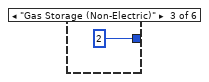
[diagram p6: hidden frame]
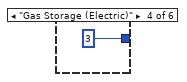
[diagram p7: hidden frame]
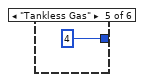
[diagram p8: hidden frame]
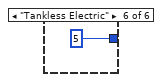
[diagram p9: hidden frame]
diagram:
  # "Elapsed Time (sec)"
  # "Take a look at this. I do not check if the water heater is heating at this point. \n\nIn preparation for determining the energy consumed during standby, record the reading given on the electrical energy (watt-hour) meter, the gas meter,\n and/or the scale used to determine oil consumption, as appropriate. Record the mean tank temperature at the start of the standby period (Tsu,0). At 1-minute\n intervals, record ambient temperature, the electric and/or fuel instrument readings, and the mean tank temperature until the next draw is initiated. The end of\n the standby period is when the final mean tank temperature is recorded, as described. Just prior to initiation of the next draw, record the mean tank temperature\n (Tsu,f). If the water heater is undergoing recovery when the next draw is initiated, record the mean tank temperature (Tsu,f) at the minute prior to the start of the\n recovery. Determine the total electrical energy and/or fossil fuel energy consumption from the beginning of the test to the end of the standby period (Qsu,f). Record\n the time interval between the start of the standby period and the end of the standby period (tstby,1).\n\n\nif the compressor comes on during this time, it is not 10 hours 29 minutes..but it is now 1 minute prior to the compressor coming on."
  # "Alan calculates this value at 37800-60 seconds. This is exactly correct. The \ndifference comes due to valve open/close in the automated sequence. It takes \napprox. 5-10 seconds. I have been reducing."
  n1 = disable-structure shown="Disabled" {
    frame Disabled {
      # "Move one step back, since\nit will overshoot by one"
      n2 = for {
        tunnel: _ -> [w27] mode=indexing
        tunnel: [w31] -> w26
        i -> [w31]
        stop <- w32 stop-if-true
        n3 = Subtract(x=37800.0 ("y"), y=60.0) -> (x-y=w28:dbl)
        n4 = Greater Or Equal?(x=w27, y=w28) -> (x >= y?=w32:bool)
      }
      n5 = Decrement(x=w26) -> ()  [unwired: 1 out]
    }
    frame Enabled {
    }
  }
  n6 = case shown="\"Standard Electric\", \"Standard Electronic\", Default" "Water Heater Type" {
    tunnel: [u8 0 u8 1 u8 2 u8 3 u8 4 u8 5] -> w17
    frame "Standard Electric", "Standard Electronic", Default {
    }
    frame "HPWH" {
    }
    frame "Gas Storage (Non-Electric)" {
    }
    frame "Gas Storage (Electric)" {
    }
    frame "Tankless Gas" {
    }
    frame "Tankless Electric" {
    }
  }
  n7 = Unbundle By Name("UEF Calculated Values") -> ("Raw Data.Test Data-Start to End DBL"=w24:dbl[][], "Raw Data.Elapsed Time Index (DBL)"=w19:i32, "Raw Data.Watt Hours -Wh Index (DBL)"=w23:i32, "Raw Data.Energy BTU Index (DBL)"=w22:i32, "Raw Data.TC Tree Avg Index (DBL)"=w21:i32, "Raw Data.Software Elapsed Time Index (DBL)"=w20:i32, "Raw Data.Heat Source Index (DBL)"=w11:i32, "Static Data.V - Volume of Wh (True)"=w8:dbl, "Data Indexes.Draws in Cluster"=w3:i32, "Data Indexes.Tsu0 Index (Found)"=w7:i32, "Data Indexes.Start Watt Hours"=w5:dbl, "Data Indexes.Start Energy (BTU-Gas)"=w4:dbl)
  n8 = disable-structure shown="Disabled" {
    frame Disabled {
      n9 = formula code="// Define variables\nuInt32 Array_Rows;\nuInt32 i;\nint32 Suf_Time;\nint32 Decrement_Time = 60;\nint32 Suf_Index = -1;  // default value in case not found\nfloat Qsuf_Electric;\nfloat Qsuf_Gas;\nfloat WH_TO_BTU = 3.41214;   // This is the conversion of Watt-Hours to BTU\nfloat End_of_Standby_Time;\n\n// Determine number of rows in Elapsed_Time array\nArray_Rows = sizeOfDim(Elapsed_Time, 0);\n\n// Determine Suf_Time based on Draw_Pattern. In the very low usage pattern, the standby end time is different.\nif (Draw_Pattern == 5) {\n    Suf_Time = 28800 - Decrement_Time;  // 8:00 hour mark - 1 minute\n    End_of_Standby_Time = 28800;             // This is the time when the draw is initiated\n} else {\n    Suf_Time = 37800 - Decrement_Time;  // 10:30 mark - 1 minute\n    End_of_Standby_Time = 37800;             // This is the time when the draw is initiated\n}\n\n// Loop forward to find first Elapsed_Time >= Suf_Time\nfor (i = 0; i < Array_Rows; i++) {\n    if (Elapsed_Time[i] >= Suf_Time) {\n        Suf_Index = i;\n        Elapsed_Time_At_Suf = Test_Data_StartToEnd[Suf_Index][Elapsed_Time_Index];\n        Software_Time_At_Suf = Test_Data_StartToEnd[Suf_Index][Software_Elapsed_Time_Index];\n        Q_Watt_Hours_Suf = Test_Data_StartToEnd[Suf_Index][Watt_Hours_Index];\n        Q_EnergyBTU_Index_Suf = Test_Data_StartToEnd[Suf_Index][EnergyBTU_Index];\n        TC_Tree_Avg_Suf = Test_Data_StartToEnd[Suf_Index][TC_Tree_Avg_Index];\n        Tau_stby_1_hr = (Software_Time_At_Suf - Software_Elapsed_Time_At_Suo)/3600;   //Time in hours between Su0 and Suf\n        break;\n    }\n}\n\n// Based on the water heater type, evaluate the Qsuf in BTU\nif (Water_Heater_Type == 0) {\n// Calculate Qsuf for Standard Electric and Standard Electronic\nQsuf = Q_Watt_Hours_Suf*WH_TO_BTU;\n}\n\nelse if (Water_Heater_Type == 1) {\n// Calculate Qsuf for HPWH\nQsuf = Q_Watt_Hours_Suf*WH_TO_BTU;\n}\n\nelse if (Water_Heater_Type == 2) {\n// Calculate Qsuf for Gas Storage (Non-Electric)\nQsuf = Q_EnergyBTU_Index_Suf;\n}\n\nelse if (Water_Heater_Type == 3) {\n// Calculate Qsuf for Gas Storage (Electric)\nQsuf_Electric = Q_Watt_Hours_Suf*WH_TO_BTU;\nQsuf_Gas = Q_EnergyBTU_Index_Suf;\n// Add the energy in BTU\nQsuf = Qsuf_Electric + Qsuf_Gas;\n}\n\nelse if (Water_Heater_Type == 4) {\n// Calculate Qsuf for Tankless Gas\nQsuf_Electric = Q_Watt_Hours_Suf*WH_TO_BTU;\nQsuf_Gas = Q_EnergyBTU_Index_Suf;\n// Add the energy in BTU\nQsuf = Qsuf_Electric + Qsuf_Gas;\n}\n\nelse if (Water_Heater_Type == 5) {\n// Calculate Qr for Tankless Electric\nQsuf = Q_Watt_Hours_Suf*WH_TO_BTU;\n}\n\nelse {\n// Default case: Invalid heater type\nQsuf = 0;\n}"() -> ()  [unwired: 12 in, 8 out]
    }
    frame Enabled {
    }
  }
  n10 = disable-structure shown="Disabled" {
    frame Disabled {
      n11 = formula code="//--------------------------------------------------------------------\n//  Tsuf, Qsuf, tstby,1   — 10 CFR 430 Appendix E (§5.4.2)\n//  • Skips standby block when Tank_Volume_Gal < 2 (flow-activated)\n//  • Works for draw patterns 1-5 (add cases if you use others)\n//--------------------------------------------------------------------\n\n//-------- LOCAL DECLARATIONS (all at top) --------------------------\nint32  i, N;\nfloat  StandbyEndGate;\nint32  Tsf_Index          = -1;      // candidate Tsuf index\nfloat WH_TO_BTU = 3.41214;\nfloat  Q_wh;\nfloat  Q_btu;\nint32 k;                 // iterator to find OFF row\nint32 m;                 // iterator to walk back 60 s\nfloat time_off;          // elapsed-time stamp at OFF row\n\n//-------- DEFAULT OUTPUTS (safe zeros) -----------------------------\nTsuf = 0.0;\nQsuf = 0.0;\nTau_stby_1_hr = 0.0;\nSoftware_Time_At_Suf = 0;\n\n//-------- BYPASS FOR < 2-GAL UNITS (no standby test) ---------------\nif (Tank_Volume_Gal >= 2.0) {\n\n    //---- 1.  Standby-end gate = 1 min (60 s) before next draw ----\n    if (Draw_Pattern == 5) {                 // Very-Low usage\n        StandbyEndGate = 28800.0 - 60.0;     // 8 h 00 m -1 min\n    } else {                                 // Patterns 1-4\n        StandbyEndGate = 37800.0 - 60.0;     // 10 h 30 m -1 min\n    }\n\n    //---- 2.  First sample = End gate, starting at Tsuo index --------\n    N = sizeOfDim(Elapsed_Time, 0);\n\n    for (i = Tsu0_Index; i < N; i++) {\n        if (Elapsed_Time[i] >= StandbyEndGate) {\n            Tsf_Index = i;\n            break;\n        }\n    }\n\n//--------------------------------------------------------------------\n// 3.  Candidate row is burner-ON ?\n//     • Walk back to the last OFF minute before recovery starts\n//     • Then walk back an additional 60 s from that OFF row\n//--------------------------------------------------------------------\nif (Tsf_Index >= 0 && Test_Data_StartToEnd[Tsf_Index][Heat_Source_Index] == 1) {\n\n    //—— 3-A.  Walk back until Heat_Source switches OFF —\n    for (k = Tsf_Index; k > 0; k--) {\n        if (Test_Data_StartToEnd[k][Heat_Source_Index] == 0) {\n            break;           // found the first OFF row\n        }\n    }\n    time_off = Elapsed_Time[k];   // elapsed-time at last OFF minute\n\n    //—— 3-B.  From that OFF row, walk back = 60 seconds —\n    for (m = k; m > 0; m--) {\n        if ((time_off - Elapsed_Time[m]) >= 60.0) {\n            break;          // reached a row = 60 s before recovery\n        }\n    }\n\n    Tsf_Index = m;          // new Tsf index per eCFR wording\n}\n\n    //---- 4.  Stamp outputs when a valid index is found -----------\n    if (Tsf_Index >= 0) {\n\n        Tsuf          = Test_Data_StartToEnd[Tsf_Index][TC_Tree_Avg_Index];\n        Q_wh          = Test_Data_StartToEnd[Tsf_Index][Watt_Hours_Index];\n        Q_btu         = Test_Data_StartToEnd[Tsf_Index][EnergyBTU_Index];\n        Tau_stby_1_hr = (Elapsed_Time[Tsf_Index] - Elapsed_Time[Tsu0_Index]) / 3600.0;\n        Software_Time_At_Suf = Test_Data_StartToEnd[Tsf_Index][Software_Elapsed_Time_Index];\n\n        //-- Convert Qsuf to Btu by heater type\n        if (Water_Heater_Type == 0 ||  // Standard electric\n            Water_Heater_Type == 1 ||  // HPWH\n            Water_Heater_Type == 5) {  // Tankless electric\n            Qsuf = Q_wh * WH_TO_BTU;\n        }\n        else if (Water_Heater_Type == 2) {  // Gas storage (no electric)\n            Qsuf = Q_btu;\n        }\n        else if (Water_Heater_Type == 3 ||  // Gas+electric storage\n                 Water_Heater_Type == 4) {  // Tankless gas  (= 2 gal buffer)\n            Qsuf = Q_btu + (Q_wh * WH_TO_BTU);\n        }\n        else {                              // Unknown type\n            Qsuf = 0.0;\n        }\n    }\n}"() -> ()  [unwired: 11 in, 8 out]
    }
    frame Enabled {
    }
  }
  n12 = Index Array(array=w24, index (col)=w19) -> (element=w6:dbl[])  [unwired: 1 in]
  n13 = formula code="//--------------------------------------------------------------------------\n//  Tsuf, Qsuf, tstby,1   — per 10 CFR 430 App E (§ 5.4.2)\n//  • Skips the 8-h standby block for flow-activated units (< 2 gal)\n//  • Draw-pattern gate times cover Patterns 1-5 (add more if needed)\n//--------------------------------------------------------------------------\n\n//-------- LOCAL DECLARATIONS ----------------------------------------------\nint32  i, k, m, N, Standby_Valid ;\nfloat  StandbyEndGate;\nint32  Tsf_Index = -1;                 // will hold the final Tsuf index\nfloat WH_TO_BTU = 3.41214;   // Convert Watt-Hours to BTU\n\nfloat  Q_wh, Q_btu;\nfloat  time_off;                // elapsed-time stamp at last OFF minute\n\n//-------- DEFAULT OUTPUTS (safe zeros) -----------------------------------\nTsuf            = 0.0;\nQsuf            = 0.0;\nTau_stby_1_hr   = 0.0;\nSoftware_Time_At_Suf = 0;\n\n//-------- BYPASS FOR < 2-GAL UNITS (no standby test) ---------------------\nif (Tank_Volume_Gal >= 2.0) {\n\n    //––– 1.  Standby-end gate = next-draw time - 60 s ––––––––––––––––––\n    switch (Draws_In_Cluster) {\n        case 5:                            // Very-Low (next draw at 8 h 00 m)\n            StandbyEndGate = 28800.0 - 60.0;\n            break;\n        default:                           // Patterns 1-4 (next draw 10 h 30 m)\n            StandbyEndGate = 37800.0 - 60.0;\n            break;\n    }\n\n//––– 2.  Locate Tsuf candidate at standby-end gate ––––––––––––––––––\n//      CFR gap case (Needs Clarification from DOE and AHRI):\n//      If post-recovery pilot heat continues to raise mean tank temperature,\n//      the Branch 2A Tsu0 maximum may occur at or beyond the standby-end gate.\n//      In that case, the first-cluster standby interval collapses\n//      (Tsuf_Index <= Tsu0_Index) and cannot be used for standby-loss\n//      calculations. Pilot-only heating is not treated as recovery.\n\nN = sizeOfDim(Elapsed_Time, 0);\n\n// Assume invalid until proven valid\nStandby_Valid = 0;\n\nif (Tsu0_Index >= 0 && Tsu0_Index < N) {\n\n    // Tsu0 must occur before the standby-end gate.\n    // Compare elapsed time, not index, to StandbyEndGate.\n    if (Elapsed_Time[Tsu0_Index] < StandbyEndGate) {\n\n        for (i = Tsu0_Index; i < N; i++) {\n            if (Elapsed_Time[i] >= StandbyEndGate) {\n                Tsf_Index = i;\n                Standby_Valid = 1;\n                break;\n            }\n        }\n    }\n}\n\n    //––– 3.  If that sample is burner-ON, adjust per eCFR wording –––––––\n    if (Tsf_Index >= 0 && Test_Data_StartToEnd[Tsf_Index][Heat_Source_Index] == 1) {\n\n        /* 3-A  Walk back through contiguous ON rows to last OFF row */\n        for (k = Tsf_Index; k > 0; k--) {\n            if (Test_Data_StartToEnd[k][Heat_Source_Index] == 0) { break; }\n        }\n        time_off = Elapsed_Time[k];\n\n        /* 3-B  From that OFF row walk back = 60 s */\n        for (m = k; m > 0; m--) {\n            if ((time_off - Elapsed_Time[m]) >= 60.0) { break; }\n        }\n        Tsf_Index = m;   // minute = 60 s before recovery begins\n    }\n   \n       //––– 3-C. Final standby-period validity check –––––––––––––––––––\n       //      Section 3 may move Tsuf backward.  After all Tsuf index\n       //      adjustments are complete, Tsuf must still occur after Tsu0.\n        if (Standby_Valid == 1) {\n            if (Tsf_Index <= Tsu0_Index) {\n                Tsf_Index = -1;\n                Standby_Valid = 0;\n            }\n        }\n\n    //––– 4.  Stamp outputs if Tsf_Index is valid ––––––––––––––––––––––––\n    if (Tsf_Index >= 0 && Standby_Valid == 1) {\n\n        Tsuf  = Test_Data_StartToEnd[Tsf_Index][TC_Tree_Avg_Index];\n        Q_wh  = (Test_Data_StartToEnd[Tsf_Index][Watt_Hours_Index])-StartWatt_Hours;\n        Q_btu = (Test_Data_StartToEnd[Tsf_Index][EnergyBTU_Index])-StartEnergyBTU_Gas;\n        Tau_stby_1_hr = (Elapsed_Time[Tsf_Index] - Elapsed_Time[Tsu0_Index]) / 3600.0;\n        Software_Time_At_Suf = Test_Data_StartToEnd[Tsf_Index][Software_Elapsed_Time_Index];\n\n        /* 4-A  Convert Qsuf to Btu by heater type */\n        if (Water_Heater_Type == 0 ||   // Std electric\n            Water_Heater_Type == 1 ||   // HPWH\n            Water_Heater_Type == 5) {   // Tankless electric\n            Qsuf = Q_wh * WH_TO_BTU;\n        }\n        else if (Water_Heater_Type == 2) {      // Gas storage, no electric\n            Qsuf = Q_btu;\n        }\n        else if (Water_Heater_Type == 3 ||      // Gas+electric storage\n                 Water_Heater_Type == 4) {      // Tankless gas (= 2 gal buffer)\n            Qsuf = Q_btu + (Q_wh * WH_TO_BTU);\n        }\n        else {                                  // Unknown type\n            Qsuf = 0.0;\n        }\n    }\n}   //—— end  = 2 gal branch ————————————————————————————————"("Elapsed_Time"=w6, "Draws_In_Cluster"=w3, "Test_Data_StartToEnd"=w24, "Watt_Hours_Index"=w23, "EnergyBTU_Index"=w22, "TC_Tree_Avg_Index"=w21, "Software_Elapsed_Time_Index"=w20, "Water_Heater_Type"=w17, "Heat_Source_Index"=w11, "Tank_Volume_Gal"=w8, "Tsu0_Index"=w7, "StartWatt_Hours"=w5, "StartEnergyBTU_Gas"=w4) -> ("Tsf_Index"=w13:i32, "Software_Time_At_Suf"=w9:dbl, "Tsuf"=w14:dbl, "Tau_stby_1_hr"=w15:dbl, "Qsuf"=w12:dbl, "Standby_Valid"=w2:i32)
  n14 = case shown="1" w2 {
    tunnel: [FALSE TRUE] -> w1
    frame 0, Default {
    }
    frame 1 {
    }
  }
  n15 = Bundle By Name(cluster="UEF Calculated Values", "Sampled Data.Tau stby_1 (hr)"=w15, "Sampled Data.T suf(°F)"=w14, "Data Indexes.Tsf Index (Found)"=w13, "Sampled Data.Qsuf (BTU)"=w12, "Data Indexes.Tsf Timestamp"=w9, "Data Indexes.Standby Valid"=w1) -> (→"UEF Calculated Values Output":T1)
  "error out" <- "error in (no error)"
